vi "20220114_00.vi"() -> ()   [LabVIEW 2019]
uses:
  <vilib>/Utility/miscctls.llb/LVRowAndColumnTypeDef.ctl
panel:
  out "Cell Position":T1
  out "Table Control":string[][](table)
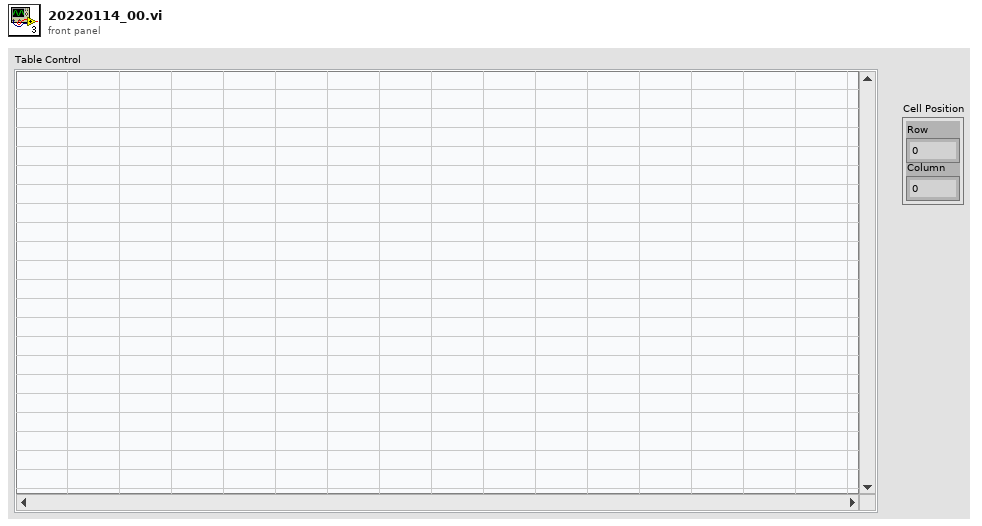
[diagram p1: front panel]
types:
  T1 = typedef "LVRowAndColumnTypeDef.ctl" = cluster{"Row":i32, "Column":i32}
  T2 = typedef "LVPoint32TypeDef.ctl" = cluster{"Horizontal":i32, "Vertical":i32}
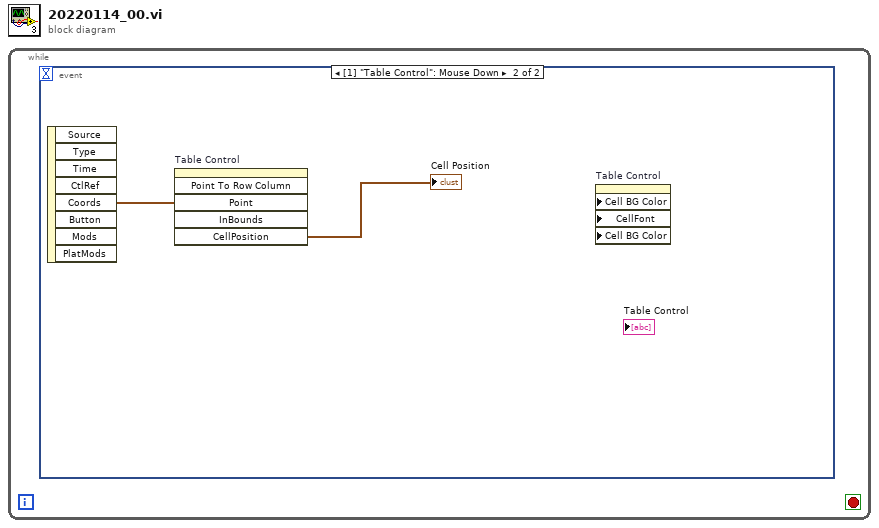
[diagram p0: block diagram]
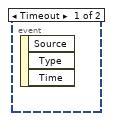
[diagram p2: hidden frame]
diagram:
  n1 = while {
    stop <- _ stop-if-true
    n2 = event shown="[1] \"Table Control\": Mouse Down" {
      selector: _ -> [_ _]
      dyn-events: _ -> [_ _]
      timeout: _ -> [_ _]
      event Timeout {
        n3 = event-data() -> ()  [unwired: 1 in, 3 out]
      }
      event "Table Control": Mouse Down {
        n4 = event-data() -> ("Coords"=w2:T2)  [unwired: 1 in, 7 out]
        n5 = invoke on="Table Control" class="Tbl (strict)" method="Point To Row Column"("Point"=w2) -> ("CellPosition"=→"Cell Position":T1)  [unwired: 5 in, 5 out]
        n6 = property on="Table Control" class="Tbl (strict)" props=["Cell BG Color", "CellFont", "Cell BG Color"]() -> ()  [unwired: 5 in, 2 out]
      }
    }
  }
